vi "Update Vehicle Position Simulation.vi"(8 "error in (no error)":errorcluster, 10 "Vehicle Pos":u32, 11 "Vehicle Position Simulation in":refnum<class "Vehicle Position Simulation.lvclass">) -> (0 "error out":errorcluster, 3 "Vehicle Position Simulation out":refnum<class "Vehicle Position Simulation.lvclass">)   [LabVIEW 2019, in "Vehicle Position Simulation.lvlib" / "Vehicle Position Simulation.lvclass"]
uses:
  Vehicle Position Simulation.lvclass
  Vehicle Position Simulation.lvclass/Vehicle Position Simulation.ctl
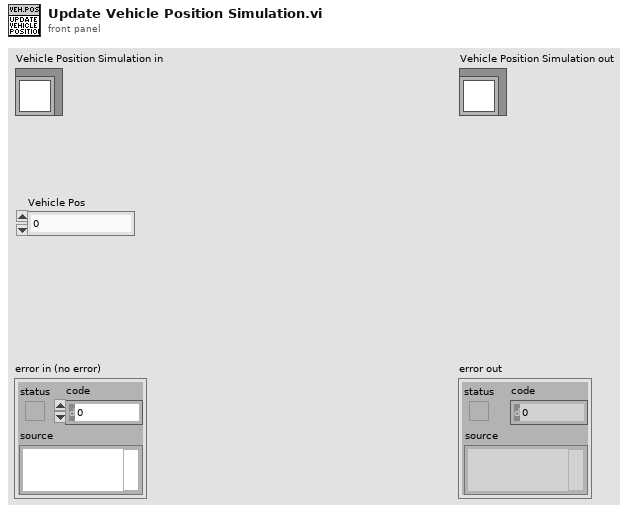
[diagram p1: front panel]
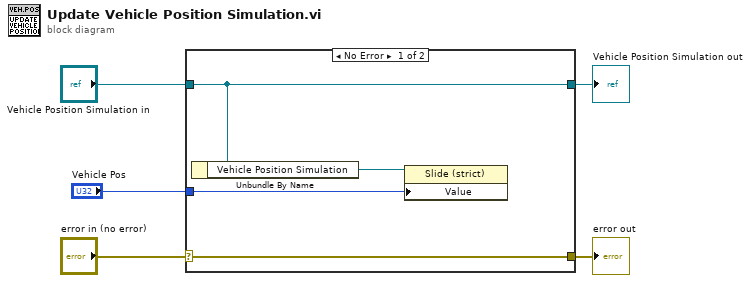
[diagram p0: block diagram]
diagram:
  n1 = case shown="No Error" "error in (no error)" {
    selector: "error in (no error)" -> [w9 w10]
    tunnel: [w9 w10] -> w4
    tunnel: [w8 w11] -> w2
    tunnel: "Vehicle Position Simulation in" -> [w8 w11]
    tunnel: "Vehicle Pos" -> [w6 _]
    frame No Error {
      n2 = Unbundle By Name(w8) -> ("Vehicle Position Simulation"=w7:refnum<vi>)
      n3 = property class="Slide (strict)"(reference=w7, "Value"=w6) -> ()  [unwired: 1 in, 2 out]
    }
    frame Error {
    }
  }
  "error out" <- w4
  "Vehicle Position Simulation out" <- w2
